vi "Linear.vi"(1 "b":T1, 2 "A":T1, 3 "W":T1) -> (0 "Z":T1)   [LabVIEW 2016]
uses:
  <vilib>/Analysis/Matrix/Datatypes/RealMatrix.ctl
  <vilib>/Analysis/Matrix/Numeric/Multiply/Multiply - RM,RM.vi
  <vilib>/Analysis/Matrix/Numeric/Add/Add - RM,RM.vi
  <vilib>/Analysis/Matrix/NI_Matrix.lvlib
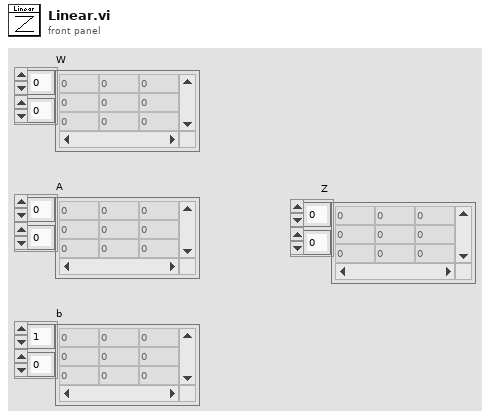
[diagram p1: front panel]
types:
  T1 = typedef "NI_Matrix.lvlib/RealMatrix.ctl" = dbl[][]
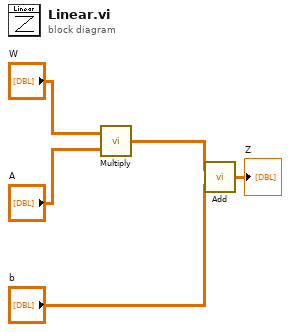
[diagram p0: block diagram]
diagram:
  n1 = call-poly <vilib>:"Multiply.vi"("Real Matrix B"="A", "Real Matrix A"="W") -> ("A * B"=w3:T1)
  n2 = call-poly <vilib>:"Add.vi"("Real Matrix B"="b", "Real Matrix A"=w3) -> ("A + B"=→"Z":T1)
